vi "Globals.vi"() -> ()   [LabVIEW 2024, in "Sift TDMS Uploader.lvlib" / "Sift TDMS Uploader.lvclass"]
uses:
  Sift TDMS Uploader.lvclass
panel:
  in  "Attribute ID":string="CSV_Export_Alias"
  # "This is used to check the global attribute manager to ensure only a single instance of this plugin is used."
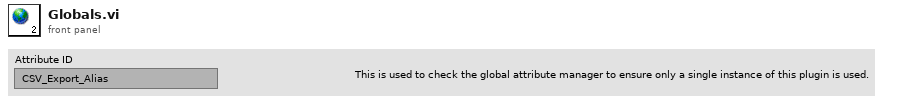
[diagram p1: front panel]
diagram:
